vi "FrameToPositions.vi"(0 "PNG Path":path, 1 "Billardbox":T2, 3 "BallDiameter":dbl=13.0, 4 "Red Range":T1={"Rmin"=91.0, "Rmax"=255.0, "Gmin"=0.0, "Gmax"=80.0, "Bmin"=0.0, "Bmax"=130.0}, 5 "Yellow Range":T1={"Rmin"=170.0, "Rmax"=255.0, "Gmin"=176.0, "Gmax"=255.0, "Bmin"=0.0, "Bmax"=175.0}, 7 "White Range":T1={"Rmin"=100.0, "Rmax"=255.0, "Gmin"=150.0, "Gmax"=255.0, "Bmin"=150.0, "Bmax"=255.0}, 9 "Range Blue Background":T1={"Rmin"=39.0, "Rmax"=62.0, "Gmin"=91.0, "Gmax"=116.0, "Bmin"=202.0, "Bmax"=255.0}, 11 "error in (no error)":errorcluster) -> (15 "error out":errorcluster, 17 "Message C / erreurs":string, 19 "Score  white":dbl, 20 "X red":dbl, 21 "Y red":dbl, 22 "Score red":dbl, 23 "X  yellow":dbl, 24 "Y  yellow":dbl, 25 "Score yellow":dbl, 26 "X  white":dbl, 27 "Y   white":dbl)   [LabVIEW 2025]
doc: "À partir d’une frame .png, ce VI : (1) lit l’image et l’affiche dans un Picture Control, (2) convertit\nl’image en fichier binaire Pixmap.bin au format attendu par le programme C, (3) exécute Pix2Pos avec les\nparamètres (BillardBox + seuils RGB + BallDiameter), (4) lit Pos.txt et extrait les positions (x,y) et scores des trois boules"
panel:
  out "standard output":string
  out "PNG picture":picture
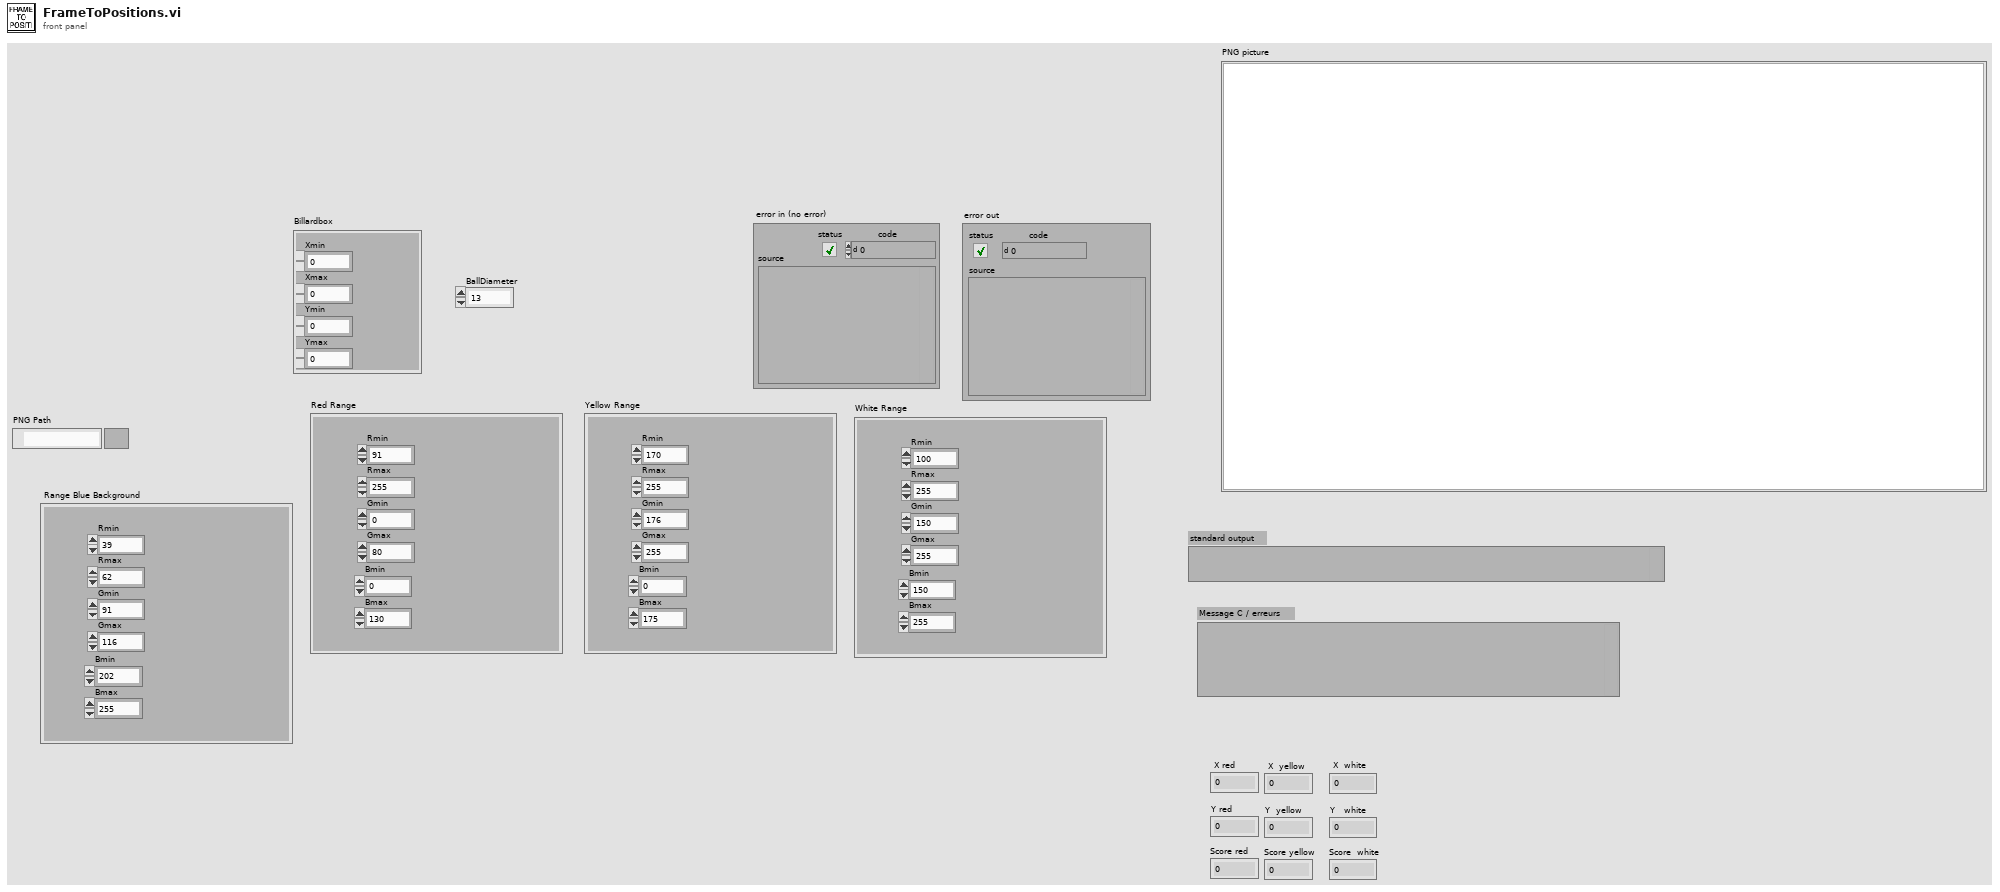
[diagram p1: front panel]
types:
  T1 = cluster{"Rmin":dbl, "Rmax":dbl, "Gmin":dbl, "Gmax":dbl, "Bmin":dbl, "Bmax":dbl}
  T2 = cluster{"Xmin":dbl, "Xmax":dbl, "Ymin":dbl, "Ymax":dbl}
  T3 = enum16{"open", "replace", "create", "open or create", "replace or create", "replace or create with confirmation"}
  T4 = enum16{"big-endian, network order", "native, host order", "little-endian"}
  T5 = typedef "imagedata.ctl" = cluster{"image type":i32, "image depth":i32, "image":u8[], "mask":u8[], "colors":u32[], "Rectangle":cluster{"left":i16, "top":i16, "right":i16, "bottom":i16}}
  T6 = cluster{"left":i16, "top":i16, "right":i16, "bottom":i16}
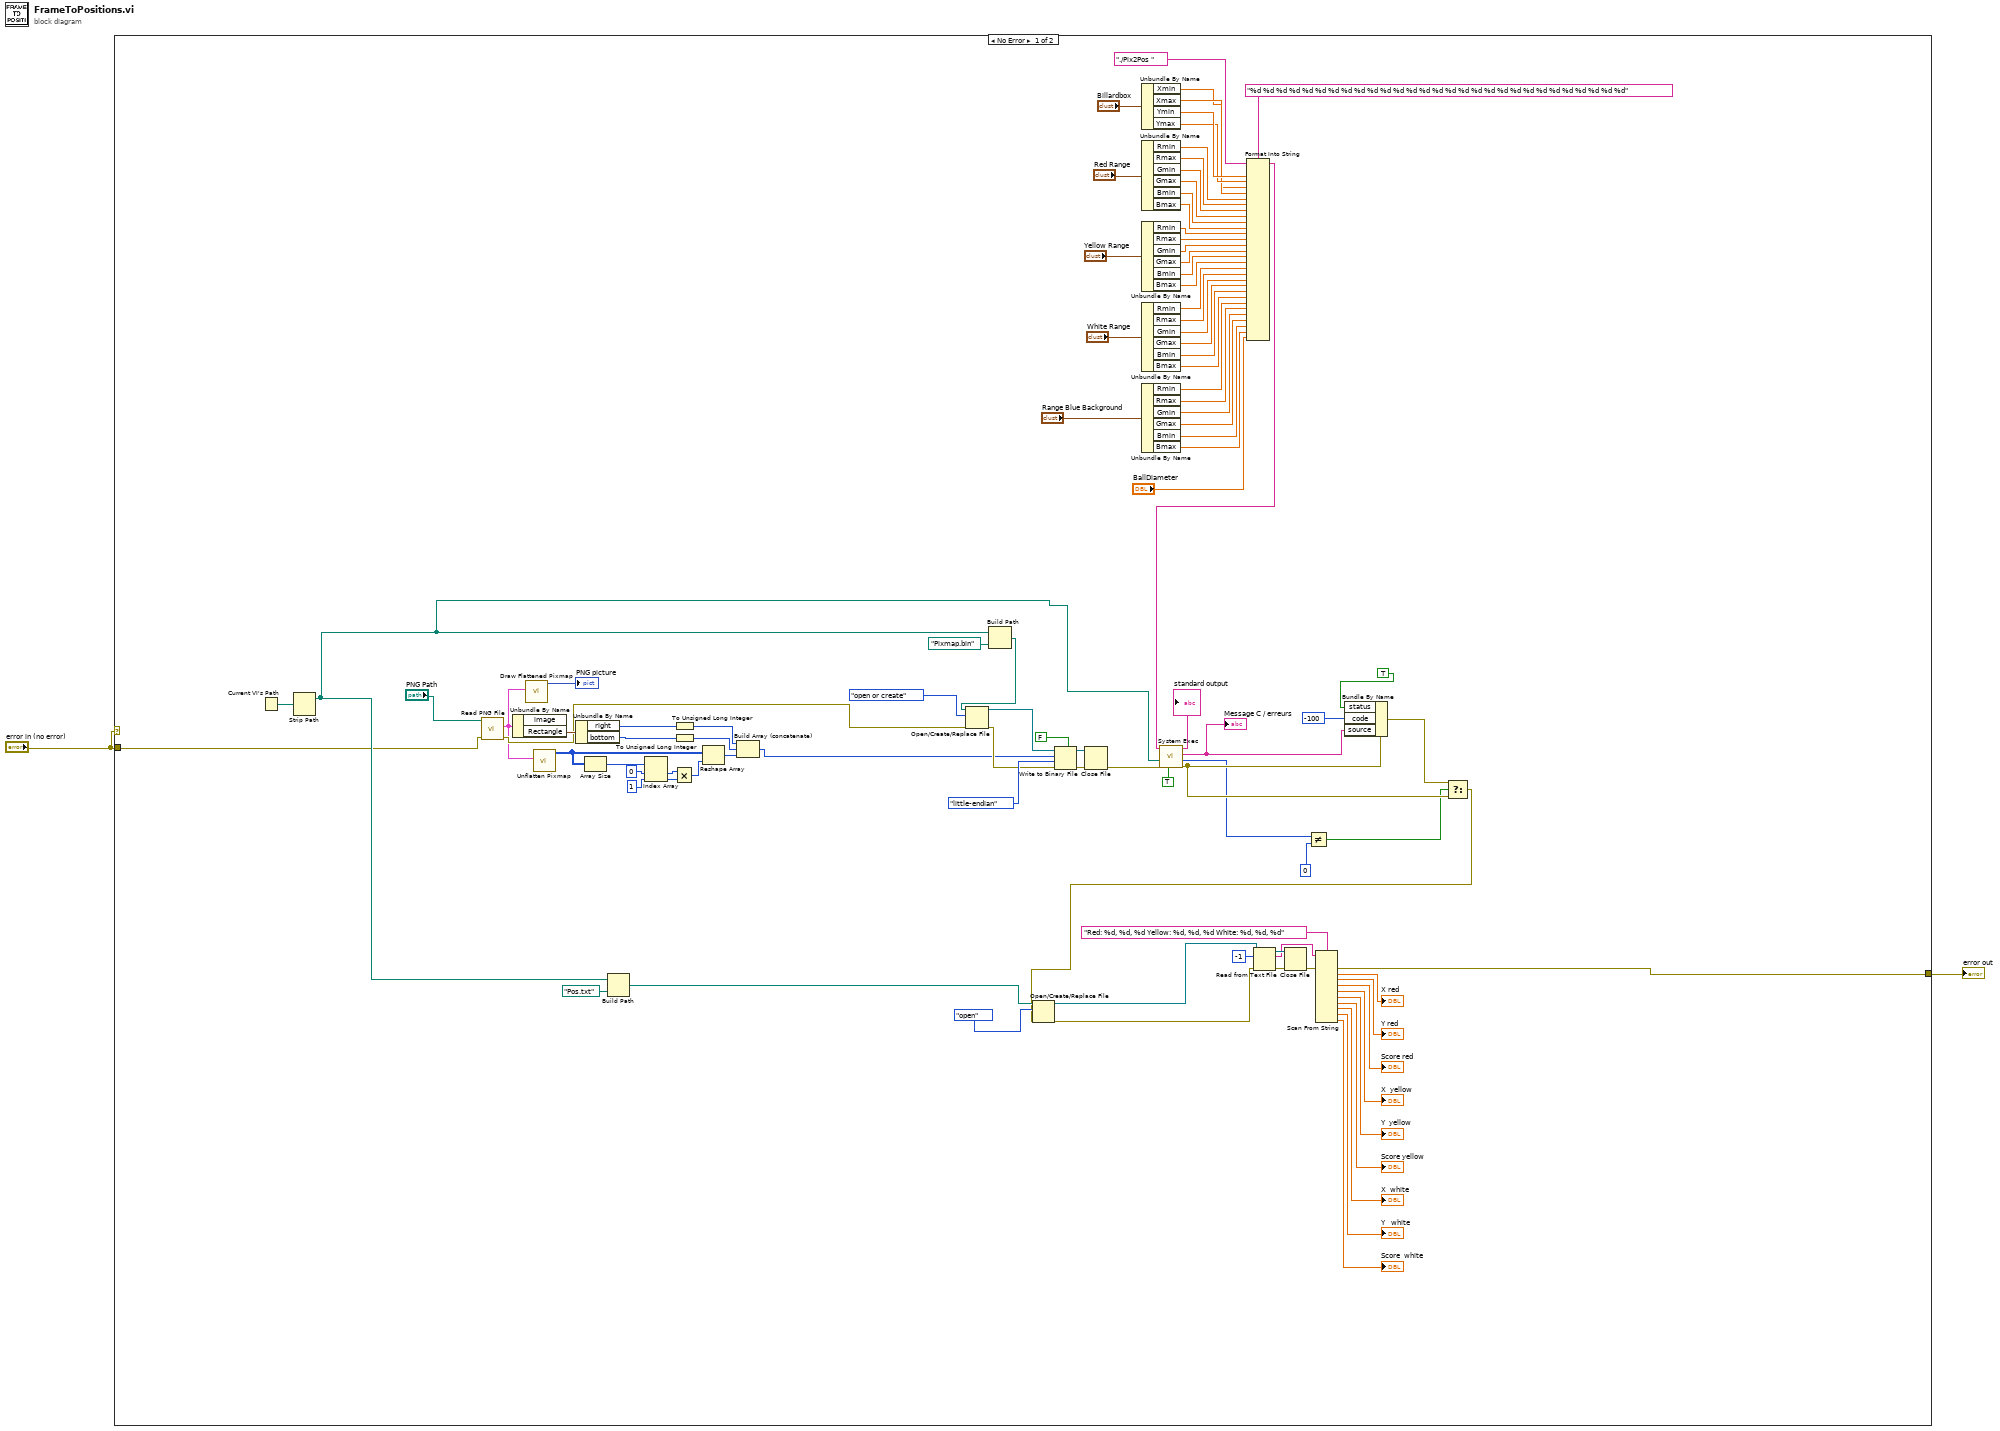
[diagram p0: block diagram]
diagram:
  n1 = case shown="No Error" "error in (no error)" {
    tunnel: "error in (no error)" -> [w22 w103]
    tunnel: [w21 w103] -> w1
    frame No Error {
      n2 = Current VI's Path() -> (path=w45:path)
      n3 = Strip Path(path=w45) -> (stripped path=w44:path)  [unwired: 1 out]
      n4 = call <vilib>:"Read PNG File.vi"("error in (no error)"=w22, "path to PNG file"="PNG Path") -> ("error out"=w57:errorcluster, "image data"=w31:T5)  [unwired: 7 in, 1 out]
      n5 = Unbundle By Name(w31) -> ("Rectangle"=w102:T6)  [unwired: 1 out]
      n6 = call <vilib>:"Draw Flattened Pixmap.vi"("image data"=w31) -> ("new picture"=→"PNG picture":picture)  [unwired: 8 in]
      n7 = call <vilib>:"Unflatten Pixmap.vi"("image data"=w31) -> ("24-bit pixmap"=w23:u32[][])  [unwired: 4 in, 6 out]
      n8 = Unbundle By Name(w102) -> ("right"=w30:i16, "bottom"=w13:i16)
      n9 = Array Size(array=w23) -> (size(s)=w29:i32[])
      n10 = Build Path(base path=w44, name or relative path=path "Pos.txt") -> (appended path=w49:path)
      n11 = Index Array(array=w29, index #1=0 ("index"), index #2=1 ("index")) -> (element #1=w26:i32, element #2=w25:i32)
      n12 = To Unsigned Long Integer(number=w30) -> (unsigned 32bit integer=w7:u32)
      n13 = To Unsigned Long Integer(number=w13) -> (unsigned 32bit integer=w12:u32)
      n14 = Multiply(x=w26, y=w25) -> (x*y=w14:i32)
      n15 = Reshape Array(w23, w14) -> (w24:u32[])
      n16 = Build Array (concatenate)(w7, w12, w24) -> (w40:u32[])
      n17 = Build Path(base path=w44, name or relative path=path "Pixmap.bin") -> (appended path=w46:path)
      n18 = Open/Create/Replace File(file path (use dialog)=w46, error in=w57, operation (0:open)=T3."open or create") -> (refnum out=w65:refnum<file>, error out=w56:errorcluster)  [unwired: 3 in, 1 out]
      n19 = Write to Binary File(file (use dialog)=w65, data=w40, error in=w56, 5:FALSE ("prepend array or string size? (T)"), 9:T4."little-endian" ("byte order (0:big-endian, network order)")) -> (refnum out=w58:refnum<file>, error out=w54:errorcluster)  [unwired: 1 in, 1 out]
      n20 = Close File(refnum=w58, error in=w54) -> (error out=w53:errorcluster)  [unwired: 1 out]
      n21 = Unbundle By Name("Billardbox") -> ("Xmin"=w3:dbl, "Xmax"=w4:dbl, "Ymin"=w6:dbl, "Ymax"=w5:dbl)
      n22 = Unbundle By Name("Red Range") -> ("Rmin"=w92:dbl, "Rmax"=w91:dbl, "Gmin"=w90:dbl, "Gmax"=w89:dbl, "Bmin"=w88:dbl, "Bmax"=w87:dbl)
      n23 = Unbundle By Name("Yellow Range") -> ("Rmin"=w86:dbl, "Rmax"=w85:dbl, "Gmin"=w84:dbl, "Gmax"=w83:dbl, "Bmin"=w82:dbl, "Bmax"=w81:dbl)
      n24 = Unbundle By Name("White Range") -> ("Rmin"=w79:dbl, "Rmax"=w78:dbl, "Gmin"=w77:dbl, "Gmax"=w76:dbl, "Bmin"=w75:dbl, "Bmax"=w74:dbl)
      n25 = Unbundle By Name("Range Blue Background") -> ("Rmin"=w72:dbl, "Rmax"=w71:dbl, "Gmin"=w70:dbl, "Gmax"=w69:dbl, "Bmin"=w68:dbl, "Bmax"=w67:dbl)
      n26 = Format Into String(format string="%d %d %d %d %d %d %d %d %d %d %d %d %d %d %d %d %d %d %d %d %d %d %d %d %d %d %d %d %d", initial string="./Pix2Pos ", w6, w5, w3, w4, w92, w91, w90, w89, w88, w87, w86, w85, w84, w83, w82, w81, w79, w78, w77, w76, w75, w74, w72, w71, w70, w69, w68, w67, "BallDiameter") -> (resulting string=w43:string)  [unwired: 1 in, 1 out]
      n27 = call <vilib>:"System Exec.vi"("run minimized? (F)"=TRUE, "error in (no error)"=w53, "working directory"=w44, "command line"=w43) -> ("error out"=w11:errorcluster, "return code"=w10:i32, "standard error"=w19:string, "standard output"=→"standard output":string)  [unwired: 4 in]
      "Message C / erreurs" <- w19
      n28 = Not Equal?(x=w10, y=0) -> (x != y?=w8:bool)
      n29 = Bundle By Name(cluster=w11, "status"=TRUE, "code"=-100, "source"=w19) -> (w17:errorcluster)
      n30 = Select(t=w17, s=w8, f=w11) -> (s? t:f=w15:errorcluster)
      n31 = Open/Create/Replace File(file path (use dialog)=w49, error in=w15, operation (0:open)=T3."open") -> (refnum out=w48:refnum<file>, error out=w55:errorcluster)  [unwired: 3 in, 1 out]
      n32 = Read from Text File(file (use dialog)=w48, count=-1, error in=w55) -> (refnum out=w64:refnum<file>, text=w52:string, error out=w62:errorcluster)  [unwired: 1 in, 1 out]
      n33 = Close File(refnum=w64, error in=w62) -> (error out=w51:errorcluster)  [unwired: 1 out]
      n34 = Scan From String(format string="Red: %d, %d, %d Yellow: %d, %d, %d White: %d, %d, %d", input string=w52, error in=w51) -> (error out=w21:errorcluster, output 1=→"X red":dbl, output 2=→"Y red":dbl, output 3=→"Score red":dbl, output 4=→"X  yellow":dbl, output 5=→"Y  yellow":dbl, output 6=→"Score yellow":dbl, output 7=→"X  white":dbl, output 8=→"Y   white":dbl, output 9=→"Score  white":dbl)  [unwired: 10 in, 2 out]
    }
    frame Error {
    }
  }
  "error out" <- w1
